vi "read-fifo.vi"(8 "FIFO In":refnum<k21>="Host_to_FPGA", 11 "numChan":i32=3) -> (2 "timout?":bool, 3 "unpacked-data":fxp<+/-,16,5>[](array[numeric]))   [LabVIEW 2017, in "FPGA-data-logging.lvlib"]
uses:
  FPGA-data-logging.lvlib
  <vilib>/rvi/DataTransferAndStorage/Container/Common/niFpgaContainerExecOnDevCompGetState.vi
  <vilib>/rvi/Emulation/niFpgaEmulationIsFPGAContextNoSignature.vi
  <vilib>/rvi/Emulation/niFpgaSctlEmulationGetInTimedLoop.vi
  <vilib>/rvi/errors/niFpgaSetErrorForExecOnDevCompSimple.vi
  <vilib>/rvi/eio/common/nirviEmuReportErrorAndStop.vi
  <vilib>/rvi/DataTransferAndStorage/Container/Common/niFpgaContainerGetUniqueNameForEmu.vi
  <vilib>/rvi/FIFO/Fifo_Resource/nirvififoEmulationSetSize.vi
  <vilib>/rvi/FIFO/Fifo_Resource/nirviFifoEmulationQueueMgr.vi
  <instcachedir>/0/nirviFifoEmulationQueueMgr_E5CAEC123FF24DC58D834DCA3CDAA9B5.lvgen/nirviFifoEmulationQueueMgr_E5CAEC123FF24DC58D834DCA3CDAA9B5_001.vi
  <vilib>/rvi/FIFO/Fifo_Resource/nirvififoEmulationDetermineInputValidOut.vi
  <vilib>/rvi/FIFO/Fifo_Resource/nirvififoEmulationCreateLock.vi
  <vilib>/rvi/Emulation/niFpgaProcessEmulError.vi
  <vilib>/rvi/FIFO/Fifo_Resource/nirvififoEmulationObtainLock.vi
  <vilib>/rvi/FIFO/Fifo_Resource/nirvififoEmulationReleaseLock.vi
  <vilib>/rvi/occurrence/nirviWaitOnOccurrenceBase.vi
  <vilib>/rvi/errors/nirviReportUnexpectedCaseInternalError.vi
  <vilib>/rvi/errors/nirviReportUnexpectedCaseInternalError (U32).vi
  <vilib>/Utility/error.llb/Clear Errors.vi
  <vilib>/rvi/interface/RandomDataEmulation/niFpgaRandomDataHandleErrors.vi
  <vilib>/rvi/DataTransferAndStorage/Container/XNode/niFpgaContainer.xnode
  <vilib>/rvi/FIFO/Fifo_Resource/niFpgaFifoEmulationRefIn.vi
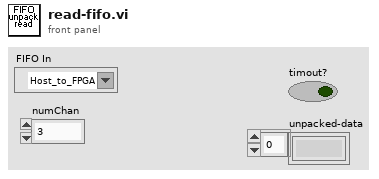
[diagram p1: front panel]
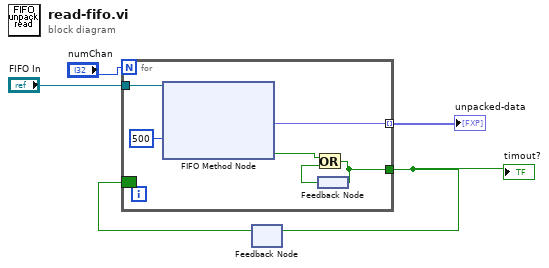
[diagram p0: block diagram]
diagram:
  n1 = feedback #1() -> (w3:bool)  [unwired: 1 in]
  n2 = for {
    N: "numChan" -> [_]
    tunnel: [w11] -> w4 mode=indexing
    tunnel: [w8] -> w5
    border: w3 -> [_]
    tunnel: "FIFO In" -> [w6]
    n3 = xnode ("FIFO Method Node")("Timeout"=500, "FIFO In"=w6) -> ("Element"=w11:fxp<+/-,16,5>, "Timed Out?"=w9:bool)  [unwired: 1 out]
    n4 = feedback #2() -> (w7:bool)
    n5 = Or(x=w9, y=w7) -> (x .or. y?=w8:bool)
    n6 = feedback-in #2(w8) -> ()
  }
  "timout?" <- w5
  "unpacked-data" <- w4
  n7 = feedback-in #1(w5) -> ()
